vi "WriteToTable.vi"(2 "引用":refnum<vi>, 3 "当前位置":string[](array[string])) -> (0 "引用输出":refnum<vi>)   [LabVIEW 2018]
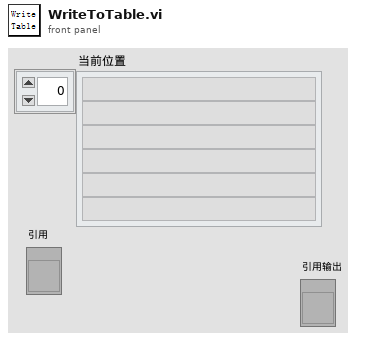
[diagram p1: front panel]
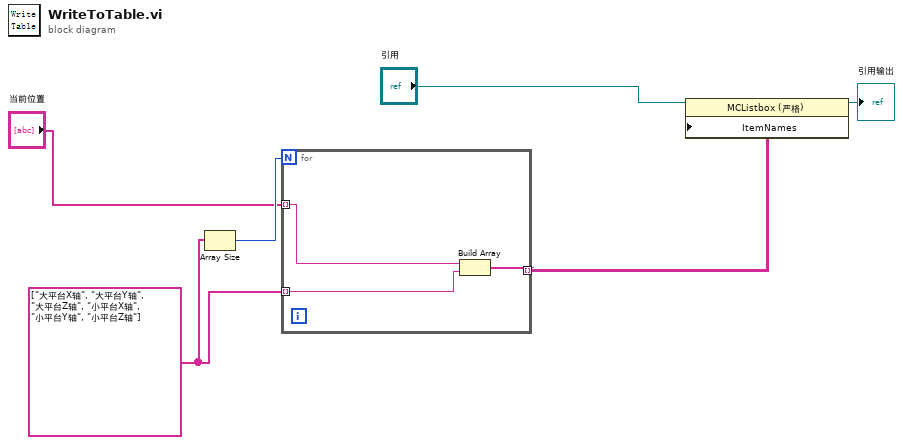
[diagram p0: block diagram]
diagram:
  w4 = string[] ["大平台X轴", "大平台Y轴", "大平台Z轴", "小平台X轴", "小平台Y轴", "小平台Z轴"]
  n1 = Array Size(array=w4) -> (size(s)=w6:i32)
  n2 = for {
    N: w6 -> [_]
    tunnel: "当前位置" -> [w9] mode=indexing
    tunnel: w4 -> [w8] mode=indexing
    tunnel: [w7] -> w2 mode=indexing
    n3 = Build Array(w9, w8) -> (w7:string[])
  }
  n4 = property on="属性节点" class="MCListbox (严格)"(reference="引用", "ItemNames"=w2) -> (reference out=→"引用输出":refnum<vi>)  [unwired: 1 in, 1 out]
